vi "报告-报警采集 - 副本.vi"   [LabVIEW 2015]
uses:
  Global control/global-1.vi
  <userlib>/_OpenG.lib/array/array.llb/Search 1D Array (Boolean)__ogtk.vi
  Global control/global-2.vi
  Global control/global-opc.vi
types:
  T1 = cluster{"Host交流故障":bool, "Host交流缺相":bool, "Host交流失电":bool, "01#JLCL交流故障":bool, "01#JLCL交流缺相":bool, "01#JLCL交流失电":bool, "02#JLCL交流故障":bool, "02#JLCL交流缺相":bool, "02#JLCL交流失电":bool, "备用1":bool, "备用2":bool, "备用3":bool, "备用4":bool, "备用5":bool, "备用6":bool, " 备用7":bool}
  T2 = cluster{"09#电源模块故障":bool, "10#电源模块故障":bool, "11#电源模块故障":bool, "12#电源模块故障":bool, "13#电源模块故障":bool, "14#电源模块故障":bool, "15#电源模块故障":bool, "16#电源模块故障":bool, "01#电源模块故障":bool, "02#电源模块故障":bool, "03#电源模块故障":bool, "04#电源模块故障":bool, "05#电源模块故障":bool, "06#电源模块故障":bool, "07#电源模块故障":bool, " 08#电源模块故障":bool}
  T3 = cluster{"09#模块通信故障":bool, "10#模块通信故障":bool, "11#模块通信故障":bool, "12#模块通信故障":bool, "13#模块通信故障":bool, "14#模块通信故障":bool, "15#模块通信故障":bool, "16#模块通信故障":bool, "01#模块通信故障":bool, "02#模块通信故障":bool, "03#模块通信故障":bool, "04#模块通信故障":bool, "05#模块通信故障":bool, "06#模块通信故障":bool, "07#模块通信故障":bool, "08#模块通信故障":bool}
  T4 = cluster{"母线过压":bool, "母线欠压":bool, "母线绝缘异常":bool, "母线绝缘预警":bool, "母线绝缘压差故障":bool, "母线交流串入故障":bool, "备用5":bool, " 备用6":bool, "电池组过压":bool, "电池组欠压":bool, "电池组过温":bool, "单体电池故障":bool, "备用1":bool, "备用2":bool, "备用3":bool, " 备用4":bool}
  T5 = cluster{"合母输出3#告警":bool, "合母输出4#告警":bool, "合母输出5#告警":bool, "合母输出6#告警":bool, "13#开关状态":bool, "14#开关状态":bool, "15#开关状态":bool, "16#开关状态":bool, "控母输出1#告警":bool, "控母输出2#告警":bool, "控母输出3#告警":bool, "控母输出4#告警":bool, "控母输出5#告警":bool, "控母输出6#告警":bool, "合母输出1#告警":bool, "合母输出2#告警":bool}
  T6 = cluster{"25#开关状态":bool, "26#开关状态":bool, "27#开关状态":bool, "28#开关状态":bool, "29#开关状态":bool, "30#开关状态":bool, "31#开关状态":bool, "32#开关状态":bool, "交流输入I告警":bool, "交流输入II告警":bool, "19#开关状态":bool, "20#开关状态":bool, "21#开关状态":bool, "22#开关状态":bool, "23#开关状态":bool, "24#开关状态":bool}
  T7 = cluster{"动作报告1":bool, "动作报告2":bool, "动作报告3":bool, "动作报告4":bool, "动作报告5":bool, "动作报告6":bool, "动作报告7":bool, "动作报告8":bool, "动作报告9":bool, "动作报告10":bool, "动作报告11":bool, "动作报告12":bool, "动作报告13":bool, "动作报告14":bool, "动作报告15":bool, "动作报告16":bool, "重合闸成功":bool, "线路测试失败":bool, "重合闸失败":bool, "手动合闸失败":bool, "一次重合":bool, "二次重合":bool, "三次重合":bool, "四次重合":bool, "失灵保护跳闸":bool, "失灵保护重跳":bool}
  T8 = cluster{"动作信号":bool, "异常告警":bool, "断路器合闸位置":bool, "隔离开关合闸位置":bool, "远方就地（1就地）":bool, "扩展板异常告警":bool, "虚遥信7":bool, "虚遥信8":bool, "虚遥信9":bool, "虚遥信10":bool, "虚遥信11":bool, "虚遥信12":bool, "虚遥信13":bool, "虚遥信14":bool, "虚遥信15":bool, "虚遥信16":bool}
  T9 = cluster{"直接合闸":bool, "分闸复位":bool, "带测合闸":bool, "MCB故障":bool, "断路器合闸反馈信号":bool, "ED储能":bool, "应急分闸":bool, "断路器分闸反馈信号":bool, "远程控制":bool, "就地控制":bool, "试验位置":bool, "工作位置":bool, "带测接触器":bool, "本站框架":bool, "邻站过流":bool, "邻站框架":bool}
  T10 = cluster{"toHMI正常运行":bool, "toHMI异常跳闸":bool, "toHMI远程":bool, "toHMI模拟中压合闸—按钮":bool, "toHMI负极柜故障报警":bool, "toHMI正极柜故障报警":bool, "toHMI馈线柜故障报警":bool, "toHMI上网柜故障报警":bool, "toHMI整流柜故障报警":bool, "toHMI压敏快熔故障":bool, "toHMI整流柜跳闸":bool, "toHMI整流柜合闸—状态":bool, "直流电流输出":u32, "直流220V电压输出":u32, "380电压输入":u32, "模拟中压合闸控制":bool, "toHMI本地":bool}
  T11 = cluster{"toHMI正常运行":bool, "toHMI设备准备好":bool, "toHMI设备异常":bool, "toHMI刀开关合—状态":bool, "toHMI刀开关分—状态":bool, "toHMI刀开关合按钮":bool, "toHMI刀开关分按钮":bool, "toHMI复位按钮":bool, "toHMI远程":bool, "toHMI本地":bool, "toHMI刀闸合—动作":bool, "toHMI刀闸分—动作":bool, "刀开关合闸控制":bool, "刀开关分闸控制":bool, "故障复位控制":bool}
  T12 = cluster{"60":bool, "70":bool, "2120":bool, "212":bool, "2121":bool, "2124":bool, "214":bool, "2140":bool, "2141":bool, "90":bool, "2110":bool, "211":bool, "2111":bool, "2113":bool, "备用1":bool, "备用2":bool}
  T13 = cluster{"toHMI正常运行":bool, "toHMI设备准备好":bool, "toHMI设备异常":bool, "toHMI高断分—状态":bool, "toHMI高断合—状态":bool, "toHMI继保故障信号":bool, "toHMI远方":bool, "toHMI本地":bool, "toHMI旁路合闸—按钮":bool, "toHMI旁路分闸—按钮":bool, "toHMI允许高断合闸—状态":bool, "toHMI旁路合分闸—状态":bool, "1500V电压输出":u32, "高断储能控制":bool, "旁路合闸控制":bool, "旁路分闸控制":bool}
  T14 = cluster{"toHMI正常运行":bool, "toHMI设备准备好":bool, "toHMI设备异常":bool, "toHMI刀开关分—状态":bool, "toHMI刀开关合—状态":bool, "toHMI框架电流故障":bool, "toHMI框架电压故障":bool, "toHMII段电压故障":bool, "toHMIII段电压故障":bool, "toHMI装置故障":bool, "toHMIMCB故障":bool, "toHMI刀开关合—完成":bool, "toHMI复位按钮":bool, "toHMI远程":bool, "toHMI本地":bool, "模拟电流框架故障控制":bool, "模拟电压框架故障控制":bool, "模拟I段电压故障控制":bool, "模拟II段电压故障控制":bool, "故障复位控制":bool}
  T15 = cluster{"toHMI刀开关合—状态":bool, "toHMI刀开关分—状态":bool, "toHMI刀开关合按钮":bool, "toHMI刀开关分按钮":bool, "toHMI远程":bool, "toHMI本地":bool, "toHMI正常运行":bool, "toHMI设备准备好":bool, "toHMI设备异常":bool, "toHMI刀闸合—动作":bool, "toHMI刀闸分—动作":bool, "toHMI接触轨有压":bool, "刀开关合闸控制":bool, "刀开关分闸控制":bool}
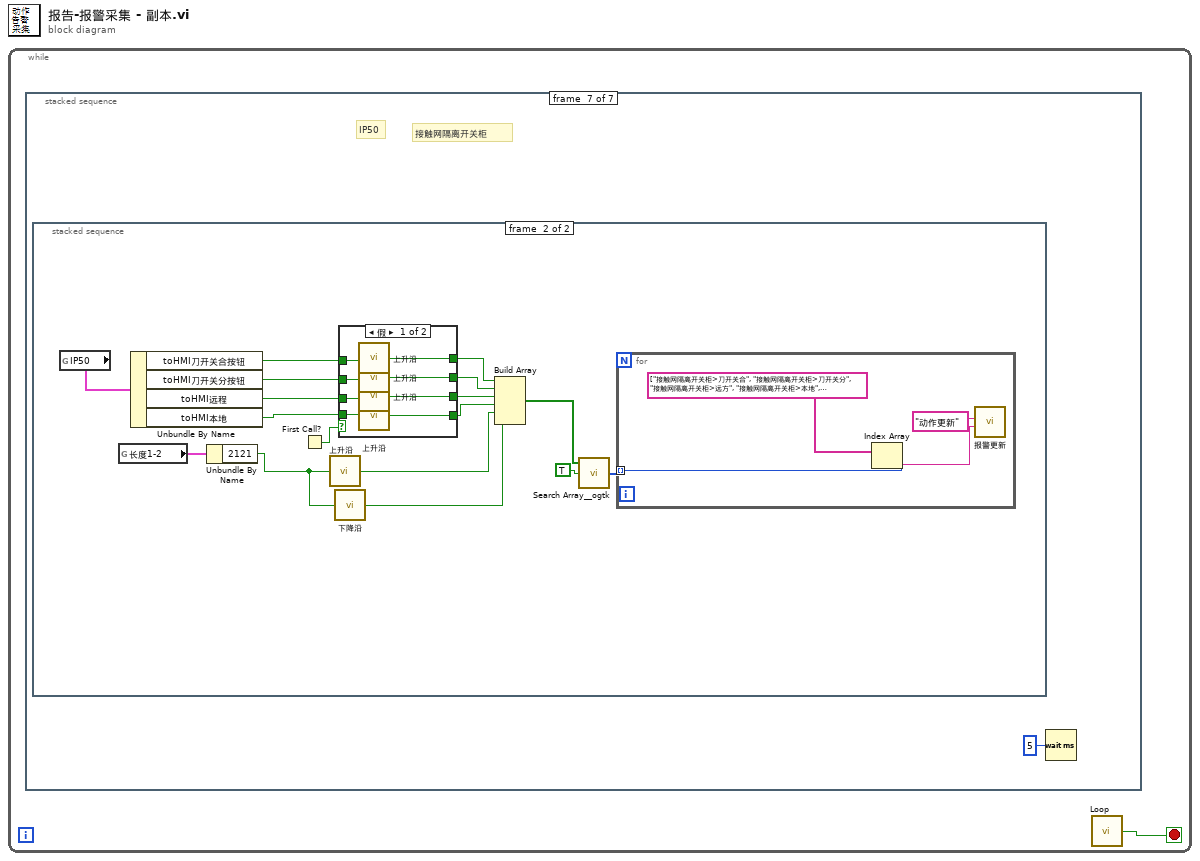
[diagram p0: block diagram]
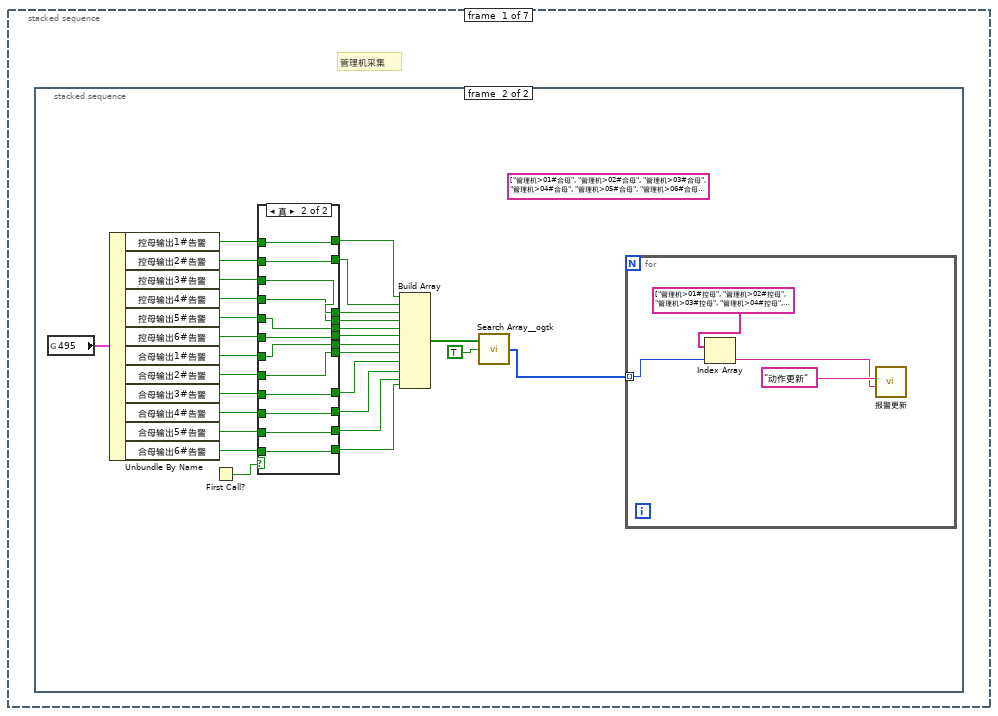
[diagram p2: hidden frame]
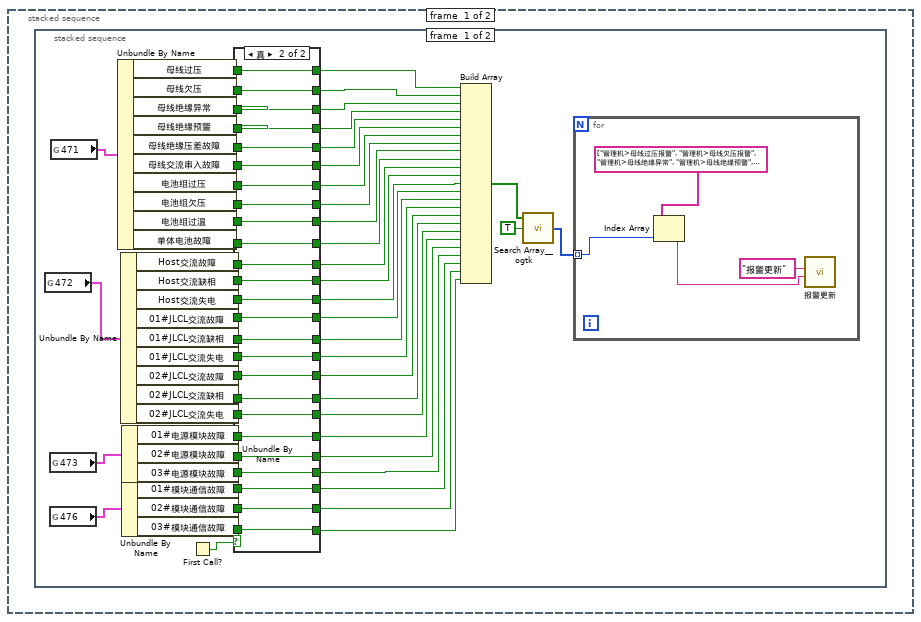
[diagram p3: hidden frame]
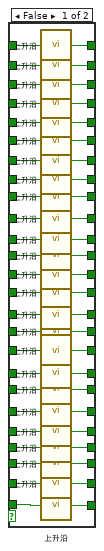
[diagram p4: hidden frame]
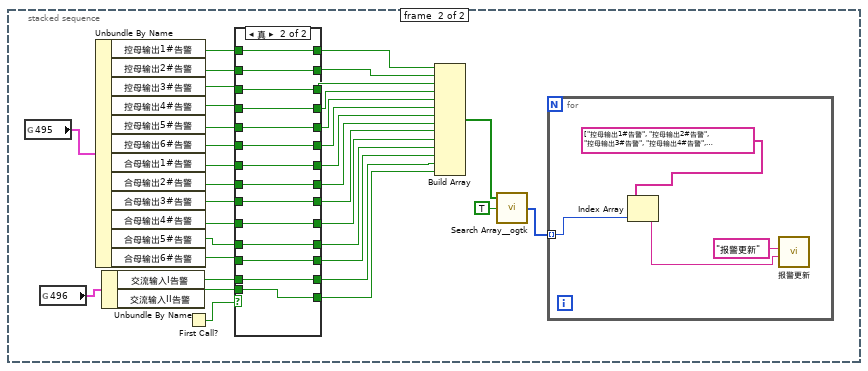
[diagram p5: hidden frame]
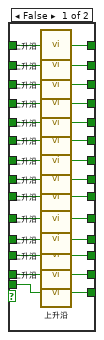
[diagram p6: hidden frame]
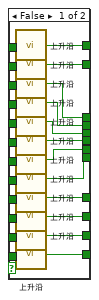
[diagram p7: hidden frame]
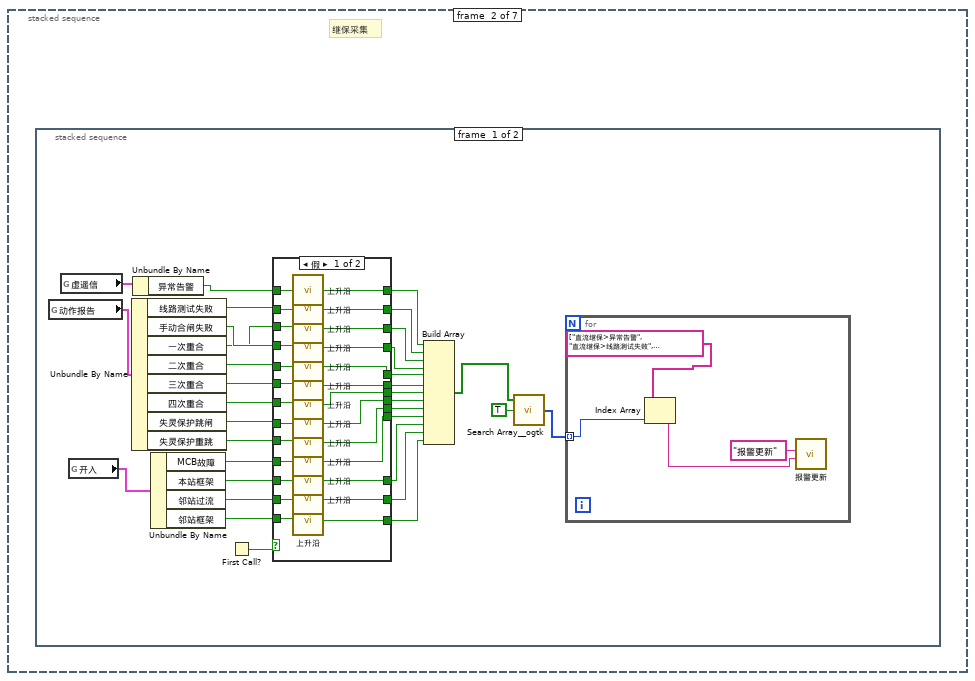
[diagram p8: hidden frame]
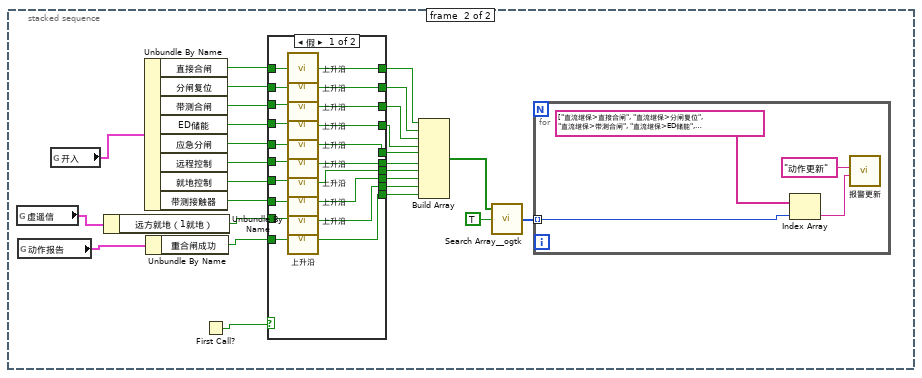
[diagram p10: hidden frame]
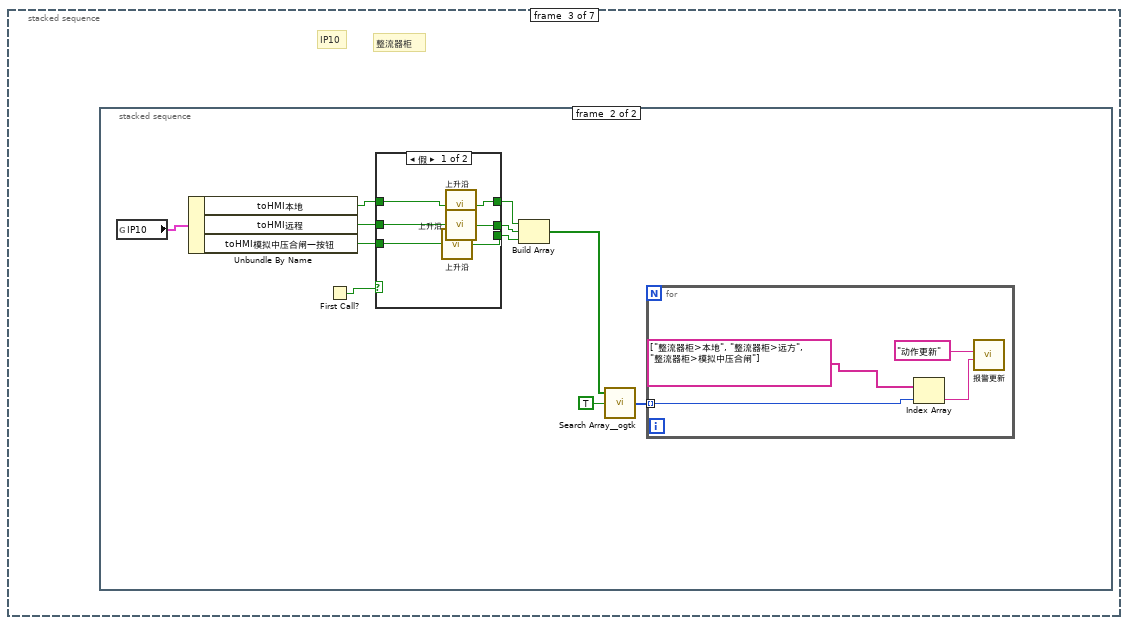
[diagram p12: hidden frame]
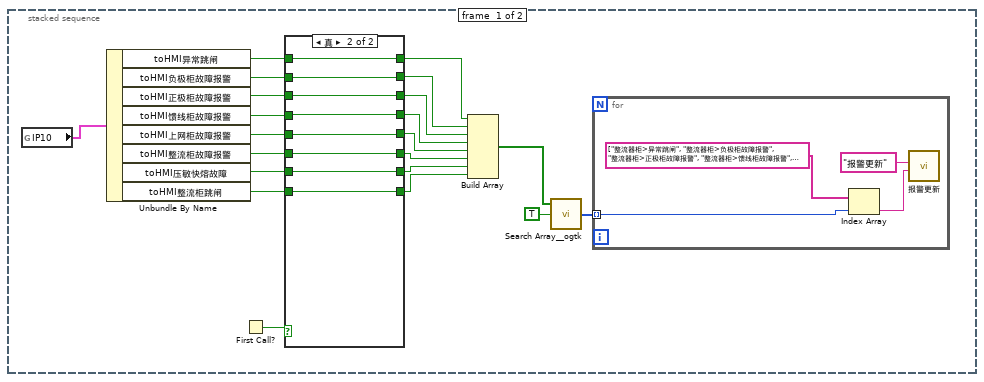
[diagram p13: hidden frame]
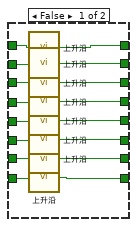
[diagram p14: hidden frame]
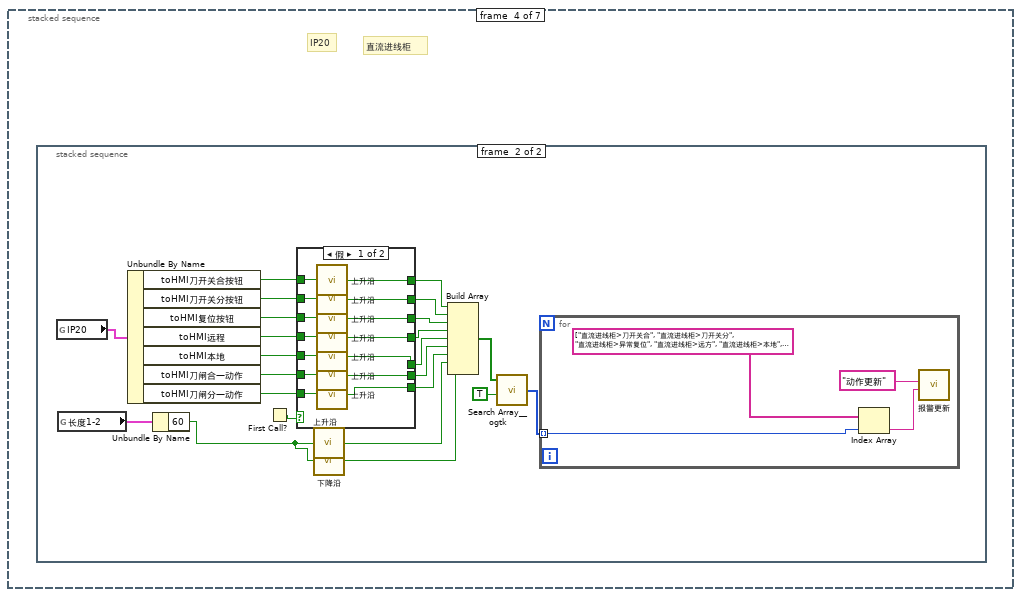
[diagram p16: hidden frame]
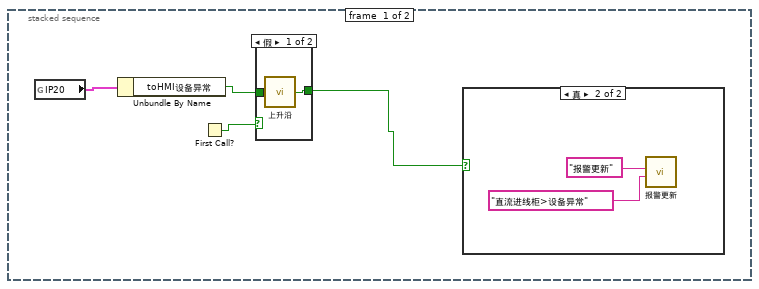
[diagram p17: hidden frame]
diagram:
  n1 = while {
    stop <- w1 stop-if-true
    n2 = stacked-sequence {
      frame #0 {
        # "管理机采集"
        n3 = stacked-sequence {
          frame #0 {
            n4 = stacked-sequence {
              frame #0 {
                n5 = global read "global-1.vi" "472"() -> (w58:T1)
                n6 = global read "global-1.vi" "473"() -> (w57:T2)
                n7 = global read "global-1.vi" "476"() -> (w56:T3)
                n8 = global read "global-1.vi" "471"() -> (w59:T4)
                n9 = Unbundle By Name(w59) -> ("母线过压"=w28:bool, "母线欠压"=w55:bool, "母线绝缘异常"=w54:bool, "母线绝缘预警"=w53:bool, "母线绝缘压差故障"=w52:bool, "母线交流串入故障"=w51:bool, "电池组过压"=w50:bool, "电池组欠压"=w49:bool, "电池组过温"=w48:bool, "单体电池故障"=w47:bool)
                n10 = Unbundle By Name(w58) -> ("Host交流故障"=w46:bool, "Host交流缺相"=w45:bool, "Host交流失电"=w44:bool, "01#JLCL交流故障"=w43:bool, "01#JLCL交流缺相"=w42:bool, "01#JLCL交流失电"=w41:bool, "02#JLCL交流故障"=w40:bool, "02#JLCL交流缺相"=w39:bool, "02#JLCL交流失电"=w38:bool)
                n11 = Unbundle By Name(w57) -> ("01#电源模块故障"=w37:bool, "02#电源模块故障"=w36:bool, "03#电源模块故障"=w35:bool)
                n12 = Unbundle By Name(w56) -> ("01#模块通信故障"=w34:bool, "02#模块通信故障"=w33:bool, "03#模块通信故障"=w32:bool)
                n13 = First Call?() -> (First Call?: T/F=w2:bool)
                n14 = case shown="真" w2 {
                  tunnel: w55 -> [w109 w133]
                  tunnel: w54 -> [w108 w132]
                  tunnel: w53 -> [w107 w131]
                  tunnel: w52 -> [w106 w130]
                  tunnel: w51 -> [w105 w129]
                  tunnel: w50 -> [w104 w128]
                  tunnel: w49 -> [w103 w127]
                  tunnel: w48 -> [w102 w126]
                  tunnel: w47 -> [w101 w125]
                  tunnel: w46 -> [w100 w124]
                  tunnel: w45 -> [w99 w123]
                  tunnel: w44 -> [w98 w122]
                  tunnel: w43 -> [w97 w121]
                  tunnel: w42 -> [w96 w120]
                  tunnel: w41 -> [w95 w119]
                  tunnel: w40 -> [w94 w118]
                  tunnel: w39 -> [w93 w117]
                  tunnel: w38 -> [w92 w116]
                  tunnel: w37 -> [w91 w115]
                  tunnel: w36 -> [w90 w114]
                  tunnel: w35 -> [w89 w113]
                  tunnel: w34 -> [w88 w112]
                  tunnel: w33 -> [w87 w111]
                  tunnel: w32 -> [w86 w110]
                  tunnel: w28 -> [w85 w134]
                  tunnel: [w84 w134] -> w27
                  tunnel: [w83 w133] -> w26
                  tunnel: [w82 w132] -> w25
                  tunnel: [w81 w131] -> w24
                  tunnel: [w80 w130] -> w23
                  tunnel: [w79 w129] -> w22
                  tunnel: [w78 w128] -> w21
                  tunnel: [w77 w127] -> w20
                  tunnel: [w76 w126] -> w19
                  tunnel: [w75 w125] -> w18
                  tunnel: [w74 w124] -> w17
                  tunnel: [w73 w123] -> w16
                  tunnel: [w72 w122] -> w15
                  tunnel: [w71 w121] -> w14
                  tunnel: [w70 w120] -> w13
                  tunnel: [w69 w118] -> w12
                  tunnel: [w68 w117] -> w11
                  tunnel: [w67 w116] -> w10
                  tunnel: [w66 w115] -> w9
                  tunnel: [w65 w114] -> w8
                  tunnel: [w64 w113] -> w7
                  tunnel: [w63 w112] -> w6
                  tunnel: [w62 w111] -> w5
                  tunnel: [w61 w110] -> w4
                  tunnel: [w60 w119] -> w3
                  frame False {
                    n15 = call "上升沿.vi"("Boolean Input"=w85) -> ("Rising Edge"=w84:bool)
                    n16 = call "上升沿.vi"("Boolean Input"=w109) -> ("Rising Edge"=w83:bool)
                    n17 = call "上升沿.vi"("Boolean Input"=w108) -> ("Rising Edge"=w82:bool)
                    n18 = call "上升沿.vi"("Boolean Input"=w107) -> ("Rising Edge"=w81:bool)
                    n19 = call "上升沿.vi"("Boolean Input"=w106) -> ("Rising Edge"=w80:bool)
                    n20 = call "上升沿.vi"("Boolean Input"=w105) -> ("Rising Edge"=w79:bool)
                    n21 = call "上升沿.vi"("Boolean Input"=w104) -> ("Rising Edge"=w78:bool)
                    n22 = call "上升沿.vi"("Boolean Input"=w103) -> ("Rising Edge"=w77:bool)
                    n23 = call "上升沿.vi"("Boolean Input"=w102) -> ("Rising Edge"=w76:bool)
                    n24 = call "上升沿.vi"("Boolean Input"=w101) -> ("Rising Edge"=w75:bool)
                    n25 = call "上升沿.vi"("Boolean Input"=w100) -> ("Rising Edge"=w74:bool)
                    n26 = call "上升沿.vi"("Boolean Input"=w99) -> ("Rising Edge"=w73:bool)
                    n27 = call "上升沿.vi"("Boolean Input"=w98) -> ("Rising Edge"=w72:bool)
                    n28 = call "上升沿.vi"("Boolean Input"=w97) -> ("Rising Edge"=w71:bool)
                    n29 = call "上升沿.vi"("Boolean Input"=w96) -> ("Rising Edge"=w70:bool)
                    n30 = call "上升沿.vi"("Boolean Input"=w95) -> ("Rising Edge"=w60:bool)
                    n31 = call "上升沿.vi"("Boolean Input"=w94) -> ("Rising Edge"=w69:bool)
                    n32 = call "上升沿.vi"("Boolean Input"=w93) -> ("Rising Edge"=w68:bool)
                    n33 = call "上升沿.vi"("Boolean Input"=w92) -> ("Rising Edge"=w67:bool)
                    n34 = call "上升沿.vi"("Boolean Input"=w91) -> ("Rising Edge"=w66:bool)
                    n35 = call "上升沿.vi"("Boolean Input"=w90) -> ("Rising Edge"=w65:bool)
                    n36 = call "上升沿.vi"("Boolean Input"=w89) -> ("Rising Edge"=w64:bool)
                    n37 = call "上升沿.vi"("Boolean Input"=w88) -> ("Rising Edge"=w63:bool)
                    n38 = call "上升沿.vi"("Boolean Input"=w87) -> ("Rising Edge"=w62:bool)
                    n39 = call "上升沿.vi"("Boolean Input"=w86) -> ("Rising Edge"=w61:bool)
                  }
                  frame True {
                  }
                }
                n40 = Build Array(w27, w26, w25, w24, w23, w22, w21, w20, w19, w18, w17, w16, w15, w14, w13, w3, w12, w11, w10, w9, w8, w7, w6, w5, w4) -> (w29:bool[])
                n41 = call-poly <userlib>:"Search Array__ogtk.vi"("Array"=w29, "Element Data"=TRUE) -> ("Indices of Elements"=w30:i32[])  [unwired: 7 in]
                n42 = for {
                  tunnel: w30 -> [w137] mode=indexing
                  n43 = Index Array(array=string[] ["管理机>母线过压报警", "管理机>母线欠压报警", "管理机>母线绝缘异常", "管理机>母线绝缘预警", "管理机>母线绝缘压差故障", "管理机>母线交流串入故障", "管理机>电池组过压", "管理机>电池组欠压", "管理机>电池组过温", "管理机>单体电池故障", "管理机>Host交流故障", "管理机>Host交流缺相", "管理机>Host交流失电", "管理机>01#JLCL交流故障", "管理机>01#JLCL交流缺相", "管理机>01#JLCL交流失电", "管理机>02#JLCL交流故障", "管理机>02#JLCL交流缺相", "管理机>02#JLCL交流失电", "管理机>01#电源模块故障", "管理机>02#电源模块故障", "管理机>03#电源模块故障", "管理机>01##模块通信故障", "管理机>02##模块通信故障", "管理机>03##模块通信故障"], index=w137) -> (element=w136:string)
                  n44 = call "报警更新.vi"("Message Data"=w136, "state"="报警更新") -> ()  [unwired: 10 in]
                }
              }
              frame #1 {
                n45 = global read "global-1.vi" "495"() -> (w172:T5)
                n46 = global read "global-1.vi" "496"() -> (w171:T6)
                n47 = Unbundle By Name(w172) -> ("控母输出1#告警"=w156:bool, "控母输出2#告警"=w170:bool, "控母输出3#告警"=w169:bool, "控母输出4#告警"=w168:bool, "控母输出5#告警"=w167:bool, "控母输出6#告警"=w166:bool, "合母输出1#告警"=w165:bool, "合母输出2#告警"=w164:bool, "合母输出3#告警"=w163:bool, "合母输出4#告警"=w162:bool, "合母输出5#告警"=w140:bool, "合母输出6#告警"=w139:bool)
                n48 = Unbundle By Name(w171) -> ("交流输入I告警"=w161:bool, "交流输入II告警"=w160:bool)
                n49 = First Call?() -> (First Call?: T/F=w141:bool)
                n50 = case shown="真" w141 {
                  tunnel: w170 -> [w200 w213]
                  tunnel: w169 -> [w199 w212]
                  tunnel: w168 -> [w198 w211]
                  tunnel: w167 -> [w197 w210]
                  tunnel: w166 -> [w196 w209]
                  tunnel: w165 -> [w195 w208]
                  tunnel: w164 -> [w194 w207]
                  tunnel: w163 -> [w193 w206]
                  tunnel: w162 -> [w192 w205]
                  tunnel: w140 -> [w191 w204]
                  tunnel: w139 -> [w190 w203]
                  tunnel: w161 -> [w189 w202]
                  tunnel: w160 -> [w188 w201]
                  tunnel: w156 -> [w187 w214]
                  tunnel: [w186 w214] -> w155
                  tunnel: [w185 w213] -> w154
                  tunnel: [w184 w212] -> w153
                  tunnel: [w183 w211] -> w152
                  tunnel: [w182 w210] -> w151
                  tunnel: [w181 w209] -> w150
                  tunnel: [w180 w208] -> w149
                  tunnel: [w179 w207] -> w148
                  tunnel: [w178 w206] -> w147
                  tunnel: [w177 w205] -> w146
                  tunnel: [w176 w204] -> w145
                  tunnel: [w175 w203] -> w144
                  tunnel: [w174 w202] -> w143
                  tunnel: [w173 w201] -> w142
                  frame False {
                    n51 = call "上升沿.vi"("Boolean Input"=w187) -> ("Rising Edge"=w186:bool)
                    n52 = call "上升沿.vi"("Boolean Input"=w200) -> ("Rising Edge"=w185:bool)
                    n53 = call "上升沿.vi"("Boolean Input"=w199) -> ("Rising Edge"=w184:bool)
                    n54 = call "上升沿.vi"("Boolean Input"=w198) -> ("Rising Edge"=w183:bool)
                    n55 = call "上升沿.vi"("Boolean Input"=w197) -> ("Rising Edge"=w182:bool)
                    n56 = call "上升沿.vi"("Boolean Input"=w196) -> ("Rising Edge"=w181:bool)
                    n57 = call "上升沿.vi"("Boolean Input"=w195) -> ("Rising Edge"=w180:bool)
                    n58 = call "上升沿.vi"("Boolean Input"=w194) -> ("Rising Edge"=w179:bool)
                    n59 = call "上升沿.vi"("Boolean Input"=w193) -> ("Rising Edge"=w178:bool)
                    n60 = call "上升沿.vi"("Boolean Input"=w192) -> ("Rising Edge"=w177:bool)
                    n61 = call "上升沿.vi"("Boolean Input"=w191) -> ("Rising Edge"=w176:bool)
                    n62 = call "上升沿.vi"("Boolean Input"=w190) -> ("Rising Edge"=w175:bool)
                    n63 = call "上升沿.vi"("Boolean Input"=w189) -> ("Rising Edge"=w174:bool)
                    n64 = call "上升沿.vi"("Boolean Input"=w188) -> ("Rising Edge"=w173:bool)
                  }
                  frame True {
                  }
                }
                n65 = Build Array(w155, w154, w153, w152, w151, w150, w149, w148, w147, w146, w145, w144, w143, w142) -> (w157:bool[])
                n66 = call-poly <userlib>:"Search Array__ogtk.vi"("Array"=w157, "Element Data"=TRUE) -> ("Indices of Elements"=w158:i32[])  [unwired: 7 in]
                n67 = for {
                  tunnel: w158 -> [w217] mode=indexing
                  n68 = Index Array(array=string[] ["控母输出1#告警", "控母输出2#告警", "控母输出3#告警", "控母输出4#告警", "控母输出5#告警", "控母输出6#告警", "合母输出1#告警", "合母输出2#告警", "合母输出3#告警", "合母输出4#告警", "合母输出5#告警", "合母输出6#告警", "交流输入I告警", "交流输入II告警"], index=w217) -> (element=w216:string)
                  n69 = call "报警更新.vi"("Message Data"=w216, "state"="报警更新") -> ()  [unwired: 10 in]
                }
              }
            }
          }
          frame #1 {
            (unwired) string[] ["管理机>01#合母", "管理机>02#合母", "管理机>03#合母", "管理机>04#合母", "管理机>05#合母", "管理机>06#合母", "管理机>01#控母", "管理机>02#控母", "管理机>03#控母", "管理机>04#控母", "管理机>05#控母", "管理机>06#控母"]
            n70 = global read "global-1.vi" "495"() -> (w235:T5)
            n71 = Unbundle By Name(w235) -> ("控母输出1#告警"=w247:bool, "控母输出2#告警"=w246:bool, "控母输出3#告警"=w245:bool, "控母输出4#告警"=w244:bool, "控母输出5#告警"=w243:bool, "控母输出6#告警"=w242:bool, "合母输出1#告警"=w241:bool, "合母输出2#告警"=w240:bool, "合母输出3#告警"=w239:bool, "合母输出4#告警"=w238:bool, "合母输出5#告警"=w237:bool, "合母输出6#告警"=w236:bool)
            n72 = First Call?() -> (First Call?: T/F=w219:bool)
            n73 = case shown="真" w219 {
              tunnel: w247 -> [w271 w283]
              tunnel: w246 -> [w270 w282]
              tunnel: w245 -> [w269 w281]
              tunnel: w244 -> [w268 w280]
              tunnel: w243 -> [w267 w279]
              tunnel: w242 -> [w266 w278]
              tunnel: w241 -> [w265 w277]
              tunnel: w240 -> [w264 w276]
              tunnel: w239 -> [w263 w275]
              tunnel: w238 -> [w262 w274]
              tunnel: w237 -> [w261 w273]
              tunnel: w236 -> [w260 w272]
              tunnel: [w259 w283] -> w234
              tunnel: [w258 w282] -> w233
              tunnel: [w257 w281] -> w232
              tunnel: [w256 w280] -> w231
              tunnel: [w255 w279] -> w230
              tunnel: [w254 w278] -> w229
              tunnel: [w253 w277] -> w228
              tunnel: [w252 w276] -> w227
              tunnel: [w251 w275] -> w226
              tunnel: [w250 w274] -> w225
              tunnel: [w249 w273] -> w224
              tunnel: [w248 w272] -> w223
              frame False {
                n74 = call "上升沿.vi"("Boolean Input"=w271) -> ("Rising Edge"=w259:bool)
                n75 = call "上升沿.vi"("Boolean Input"=w270) -> ("Rising Edge"=w258:bool)
                n76 = call "上升沿.vi"("Boolean Input"=w269) -> ("Rising Edge"=w257:bool)
                n77 = call "上升沿.vi"("Boolean Input"=w268) -> ("Rising Edge"=w256:bool)
                n78 = call "上升沿.vi"("Boolean Input"=w267) -> ("Rising Edge"=w255:bool)
                n79 = call "上升沿.vi"("Boolean Input"=w266) -> ("Rising Edge"=w254:bool)
                n80 = call "上升沿.vi"("Boolean Input"=w265) -> ("Rising Edge"=w253:bool)
                n81 = call "上升沿.vi"("Boolean Input"=w264) -> ("Rising Edge"=w252:bool)
                n82 = call "上升沿.vi"("Boolean Input"=w263) -> ("Rising Edge"=w251:bool)
                n83 = call "上升沿.vi"("Boolean Input"=w262) -> ("Rising Edge"=w250:bool)
                n84 = call "上升沿.vi"("Boolean Input"=w261) -> ("Rising Edge"=w249:bool)
                n85 = call "上升沿.vi"("Boolean Input"=w260) -> ("Rising Edge"=w248:bool)
              }
              frame True {
              }
            }
            n86 = Build Array(w234, w233, w232, w231, w230, w229, w228, w227, w226, w225, w224, w223) -> (w222:bool[])
            n87 = call-poly <userlib>:"Search Array__ogtk.vi"("Array"=w222, "Element Data"=TRUE) -> ("Indices of Elements"=w220:i32[])  [unwired: 7 in]
            n88 = for {
              tunnel: w220 -> [w286] mode=indexing
              n89 = Index Array(array=string[] ["管理机>01#控母", "管理机>02#控母", "管理机>03#控母", "管理机>04#控母", "管理机>05#控母", "管理机>06#控母", "管理机>01#合母", "管理机>02#合母", "管理机>03#合母", "管理机>04#合母", "管理机>05#合母", "管理机>06#合母"], index=w286) -> (element=w285:string)
              n90 = call "报警更新.vi"("Message Data"=w285, "state"="动作更新") -> ()  [unwired: 10 in]
            }
          }
        }
      }
      frame #1 {
        # "继保采集"
        n91 = stacked-sequence {
          frame #0 {
            n92 = global read "global-2.vi" "动作报告"() -> (w319:T7)
            n93 = global read "global-2.vi" "虚遥信"() -> (w320:T8)
            n94 = global read "global-2.vi" "开入"() -> (w318:T9)
            n95 = Unbundle By Name(w319) -> ("线路测试失败"=w304:bool, "手动合闸失败"=w289:bool, "一次重合"=w288:bool, "二次重合"=w303:bool, "三次重合"=w302:bool, "四次重合"=w301:bool, "失灵保护跳闸"=w300:bool, "失灵保护重跳"=w299:bool)
            n96 = Unbundle By Name(w320) -> ("异常告警"=w305:bool)
            n97 = Unbundle By Name(w318) -> ("MCB故障"=w298:bool, "本站框架"=w297:bool, "邻站过流"=w296:bool, "邻站框架"=w295:bool)
            n98 = First Call?() -> (First Call?: T/F=w293:bool)
            n99 = case shown="假" w293 {
              tunnel: [w350 w363] -> w317
              tunnel: [w349 w362] -> w316
              tunnel: [w348 w361] -> w315
              tunnel: [w347 w360] -> w314
              tunnel: [w346 w359] -> w313
              tunnel: [w345 w358] -> w312
              tunnel: [w344 w357] -> w311
              tunnel: [w343 w356] -> w310
              tunnel: [w342 w355] -> w309
              tunnel: [w341 w354] -> w308
              tunnel: [w340 w353] -> w307
              tunnel: [w339 w352] -> w306
              tunnel: w305 -> [w338 w363]
              tunnel: w304 -> [w337 w362]
              tunnel: w288 -> [w336 w361]
              tunnel: w289 -> [w335 w360]
              tunnel: w303 -> [w334 w359]
              tunnel: w302 -> [w333 w358]
              tunnel: w301 -> [w332 w357]
              tunnel: w300 -> [w331 w356]
              tunnel: w299 -> [w330 w355]
              tunnel: w298 -> [w329 w354]
              tunnel: w297 -> [w328 w353]
              tunnel: w296 -> [w327 w352]
              tunnel: w295 -> [w326 w351]
              tunnel: [w325 w351] -> w294
              frame False {
                n100 = call "上升沿.vi"("Boolean Input"=w338) -> ("Rising Edge"=w350:bool)
                n101 = call "上升沿.vi"("Boolean Input"=w337) -> ("Rising Edge"=w349:bool)
                n102 = call "上升沿.vi"("Boolean Input"=w336) -> ("Rising Edge"=w348:bool)
                n103 = call "上升沿.vi"("Boolean Input"=w335) -> ("Rising Edge"=w347:bool)
                n104 = call "上升沿.vi"("Boolean Input"=w334) -> ("Rising Edge"=w346:bool)
                n105 = call "上升沿.vi"("Boolean Input"=w333) -> ("Rising Edge"=w345:bool)
                n106 = call "上升沿.vi"("Boolean Input"=w332) -> ("Rising Edge"=w344:bool)
                n107 = call "上升沿.vi"("Boolean Input"=w331) -> ("Rising Edge"=w343:bool)
                n108 = call "上升沿.vi"("Boolean Input"=w330) -> ("Rising Edge"=w342:bool)
                n109 = call "上升沿.vi"("Boolean Input"=w329) -> ("Rising Edge"=w341:bool)
                n110 = call "上升沿.vi"("Boolean Input"=w328) -> ("Rising Edge"=w340:bool)
                n111 = call "上升沿.vi"("Boolean Input"=w327) -> ("Rising Edge"=w339:bool)
                n112 = call "上升沿.vi"("Boolean Input"=w326) -> ("Rising Edge"=w325:bool)
              }
              frame True {
              }
            }
            n113 = Build Array(w317, w316, w315, w314, w313, w312, w311, w310, w309, w308, w307, w306, w294) -> (w290:bool[])
            n114 = call-poly <userlib>:"Search Array__ogtk.vi"("Array"=w290, "Element Data"=TRUE) -> ("Indices of Elements"=w291:i32[])  [unwired: 7 in]
            n115 = for {
              tunnel: w291 -> [w323] mode=indexing
              n116 = Index Array(array=string[] ["直流继保>异常告警", "直流继保>线路测试失败", "直流继保>手动合闸失败", "直流继保>一次重合", "直流继保>二次重合", "直流继保>三次重合", "直流继保>四次重合", "直流继保>失灵保护跳闸", "直流继保>失灵保护重跳", "直流继保>MCB故障", "直流继保>本站框架", "直流继保>邻站过流", "直流继保>邻站框架"], index=w323) -> (element=w322:string)
              n117 = call "报警更新.vi"("Message Data"=w322, "state"="报警更新") -> ()  [unwired: 10 in]
            }
          }
          frame #1 {
            n118 = global read "global-2.vi" "虚遥信"() -> (w389:T8)
            n119 = global read "global-2.vi" "动作报告"() -> (w388:T7)
            n120 = global read "global-2.vi" "开入"() -> (w390:T9)
            n121 = Unbundle By Name(w389) -> ("远方就地（1就地）"=w369:bool)
            n122 = Unbundle By Name(w390) -> ("直接合闸"=w377:bool, "分闸复位"=w376:bool, "带测合闸"=w375:bool, "ED储能"=w374:bool, "应急分闸"=w373:bool, "远程控制"=w372:bool, "就地控制"=w371:bool, "带测接触器"=w370:bool)
            n123 = Unbundle By Name(w388) -> ("重合闸成功"=w368:bool)
            n124 = First Call?() -> (First Call?: T/F=w364:bool)
            n125 = case shown="假" w364 {
              tunnel: [w414 w424] -> w378
              tunnel: [w413 w423] -> w379
              tunnel: [w412 w422] -> w380
              tunnel: [w411 w421] -> w381
              tunnel: [w410 w420] -> w382
              tunnel: [w409 w419] -> w383
              tunnel: [w408 w418] -> w384
              tunnel: [w407 w417] -> w385
              tunnel: [w406 w416] -> w386
              tunnel: [w405 w415] -> w387
              tunnel: w377 -> [w404 w424]
              tunnel: w376 -> [w403 w423]
              tunnel: w375 -> [w402 w422]
              tunnel: w374 -> [w401 w421]
              tunnel: w373 -> [w400 w420]
              tunnel: w372 -> [w399 w419]
              tunnel: w371 -> [w398 w418]
              tunnel: w370 -> [w397 w417]
              tunnel: w369 -> [w396 w416]
              tunnel: w368 -> [w395 w415]
              frame False {
                n126 = call "上升沿.vi"("Boolean Input"=w404) -> ("Rising Edge"=w414:bool)
                n127 = call "上升沿.vi"("Boolean Input"=w403) -> ("Rising Edge"=w413:bool)
                n128 = call "上升沿.vi"("Boolean Input"=w402) -> ("Rising Edge"=w412:bool)
                n129 = call "上升沿.vi"("Boolean Input"=w401) -> ("Rising Edge"=w411:bool)
                n130 = call "上升沿.vi"("Boolean Input"=w400) -> ("Rising Edge"=w410:bool)
                n131 = call "上升沿.vi"("Boolean Input"=w399) -> ("Rising Edge"=w409:bool)
                n132 = call "上升沿.vi"("Boolean Input"=w398) -> ("Rising Edge"=w408:bool)
                n133 = call "上升沿.vi"("Boolean Input"=w397) -> ("Rising Edge"=w407:bool)
                n134 = call "上升沿.vi"("Boolean Input"=w396) -> ("Rising Edge"=w406:bool)
                n135 = call "上升沿.vi"("Boolean Input"=w395) -> ("Rising Edge"=w405:bool)
              }
              frame True {
              }
            }
            n136 = Build Array(w378, w379, w380, w381, w382, w383, w384, w385, w386, w387) -> (w365:bool[])
            n137 = call-poly <userlib>:"Search Array__ogtk.vi"("Array"=w365, "Element Data"=TRUE) -> ("Indices of Elements"=w366:i32[])  [unwired: 7 in]
            n138 = for {
              tunnel: w366 -> [w393] mode=indexing
              n139 = Index Array(array=string[] ["直流继保>直接合闸", "直流继保>分闸复位", "直流继保>带测合闸", "直流继保>ED储能", "直流继保>应急分闸", "直流继保>远方", "直流继保>本地", "直流继保>带测接触器", "直流继保>远方就地（1就地）", "直流继保>重合闸成功"], index=w393) -> (element=w392:string)
              n140 = call "报警更新.vi"("Message Data"=w392, "state"="动作更新") -> ()  [unwired: 10 in]
            }
          }
        }
      }
      frame #2 {
        # "整流器柜"
        # "IP10"
        n141 = stacked-sequence {
          frame #0 {
            n142 = global read "global-opc.vi" "IP10"() -> (w445:T10)
            n143 = Unbundle By Name(w445) -> ("toHMI异常跳闸"=w426:bool, "toHMI负极柜故障报警"=w436:bool, "toHMI正极柜故障报警"=w435:bool, "toHMI馈线柜故障报警"=w434:bool, "toHMI上网柜故障报警"=w433:bool, "toHMI整流柜故障报警"=w432:bool, "toHMI压敏快熔故障"=w431:bool, "toHMI整流柜跳闸"=w430:bool)
            n144 = First Call?() -> (First Call?: T/F=w444:bool)
            n145 = case shown="真" w444 {
              tunnel: [w465 w473] -> w437
              tunnel: [w452 w472] -> w438
              tunnel: [w464 w471] -> w439
              tunnel: [w463 w470] -> w440
              tunnel: [w462 w469] -> w441
              tunnel: [w461 w468] -> w442
              tunnel: [w460 w467] -> w443
              tunnel: w436 -> [w459 w473]
              tunnel: w435 -> [w458 w472]
              tunnel: w434 -> [w457 w471]
              tunnel: w433 -> [w456 w470]
              tunnel: w432 -> [w455 w469]
              tunnel: w431 -> [w454 w468]
              tunnel: w430 -> [w453 w467]
              tunnel: w426 -> [w451 w466]
              tunnel: [w450 w466] -> w425
              frame False {
                n146 = call "上升沿.vi"("Boolean Input"=w451) -> ("Rising Edge"=w450:bool)
                n147 = call "上升沿.vi"("Boolean Input"=w459) -> ("Rising Edge"=w465:bool)
                n148 = call "上升沿.vi"("Boolean Input"=w458) -> ("Rising Edge"=w452:bool)
                n149 = call "上升沿.vi"("Boolean Input"=w457) -> ("Rising Edge"=w464:bool)
                n150 = call "上升沿.vi"("Boolean Input"=w456) -> ("Rising Edge"=w463:bool)
                n151 = call "上升沿.vi"("Boolean Input"=w455) -> ("Rising Edge"=w462:bool)
                n152 = call "上升沿.vi"("Boolean Input"=w454) -> ("Rising Edge"=w461:bool)
                n153 = call "上升沿.vi"("Boolean Input"=w453) -> ("Rising Edge"=w460:bool)
              }
              frame True {
              }
            }
            n154 = Build Array(w425, w437, w438, w439, w440, w441, w442, w443) -> (w427:bool[])
            n155 = call-poly <userlib>:"Search Array__ogtk.vi"("Array"=w427, "Element Data"=TRUE) -> ("Indices of Elements"=w428:i32[])  [unwired: 7 in]
            n156 = for {
              tunnel: w428 -> [w448] mode=indexing
              n157 = Index Array(array=string[] ["整流器柜>异常跳闸", "整流器柜>负极柜故障报警", "整流器柜>正极柜故障报警", "整流器柜>馈线柜故障报警", "整流器柜>隔离开关柜故障报警", "整流器柜>故障报警", "整流器柜>压敏快熔故障", "整流器柜>跳闸"], index=w448) -> (element=w447:string)
              n158 = call "报警更新.vi"("Message Data"=w447, "state"="报警更新") -> ()  [unwired: 10 in]
            }
          }
          frame #1 {
            n159 = global read "global-opc.vi" "IP10"() -> (w484:T10)
            n160 = Unbundle By Name(w484) -> ("toHMI本地"=w474:bool, "toHMI远程"=w482:bool, "toHMI模拟中压合闸—按钮"=w483:bool)
            n161 = First Call?() -> (First Call?: T/F=w476:bool)
            n162 = case shown="假" w476 {
              tunnel: w483 -> [w490 w493]
              tunnel: w482 -> [w487 w492]
              tunnel: [w489 w492] -> w481
              tunnel: [w488 w493] -> w480
              tunnel: [w485 w491] -> w475
              tunnel: w474 -> [w486 w491]
              frame False {
                n163 = call "上升沿.vi"("Boolean Input"=w490) -> ("Rising Edge"=w488:bool)
                n164 = call "上升沿.vi"("Boolean Input"=w486) -> ("Rising Edge"=w485:bool)
                n165 = call "上升沿.vi"("Boolean Input"=w487) -> ("Rising Edge"=w489:bool)
              }
              frame True {
              }
            }
            n166 = Build Array(w475, w481, w480) -> (w477:bool[])
            n167 = call-poly <userlib>:"Search Array__ogtk.vi"("Array"=w477, "Element Data"=TRUE) -> ("Indices of Elements"=w478:i32[])  [unwired: 7 in]
            n168 = for {
              tunnel: w478 -> [w496] mode=indexing
              n169 = Index Array(array=string[] ["整流器柜>本地", "整流器柜>远方", "整流器柜>模拟中压合闸"], index=w496) -> (element=w495:string)
              n170 = call "报警更新.vi"("Message Data"=w495, "state"="动作更新") -> ()  [unwired: 10 in]
            }
          }
        }
      }
      frame #3 {
        # "直流进线柜"
        # "IP20"
        n171 = stacked-sequence {
          frame #0 {
            n172 = global read "global-opc.vi" "IP20"() -> (w501:T11)
            n173 = Unbundle By Name(w501) -> ("toHMI设备异常"=w500:bool)
            n174 = First Call?() -> (First Call?: T/F=w499:bool)
            n175 = case shown="假" w499 {
              tunnel: w500 -> [w505 w506]
              tunnel: [w504 w506] -> w498
              frame False {
                n176 = call "上升沿.vi"("Boolean Input"=w505) -> ("Rising Edge"=w504:bool)
              }
              frame True {
              }
            }
            n177 = case shown="真" w498 {
              frame False {
              }
              frame True {
                n178 = call "报警更新.vi"("Message Data"="直流进线柜>设备异常" ("字符串"), "state"="报警更新") -> ()  [unwired: 10 in]
              }
            }
          }
          frame #1 {
            n179 = global read "global-opc.vi" "IP20"() -> (w529:T11)
            n180 = global read "global-1.vi" "长度1-2"() -> (w510:T12)
            n181 = Unbundle By Name(w529) -> ("toHMI刀开关合按钮"=w518:bool, "toHMI刀开关分按钮"=w517:bool, "toHMI复位按钮"=w516:bool, "toHMI远程"=w515:bool, "toHMI本地"=w514:bool, "toHMI刀闸合—动作"=w513:bool, "toHMI刀闸分—动作"=w512:bool)
            n182 = Unbundle By Name(w510) -> ("60"=w509:bool)
            n183 = First Call?() -> (First Call?: T/F=w526:bool)
            n184 = case shown="假" w526 {
              tunnel: [w543 w550] -> w519
              tunnel: [w542 w549] -> w520
              tunnel: [w541 w548] -> w521
              tunnel: [w540 w547] -> w522
              tunnel: [w539 w546] -> w523
              tunnel: [w538 w545] -> w524
              tunnel: [w537 w544] -> w525
              tunnel: w518 -> [w536 w550]
              tunnel: w517 -> [w535 w549]
              tunnel: w516 -> [w534 w548]
              tunnel: w515 -> [w533 w547]
              tunnel: w514 -> [w532 w546]
              tunnel: w513 -> [w531 w545]
              tunnel: w512 -> [w530 w544]
              frame False {
                n185 = call "上升沿.vi"("Boolean Input"=w536) -> ("Rising Edge"=w543:bool)
                n186 = call "上升沿.vi"("Boolean Input"=w535) -> ("Rising Edge"=w542:bool)
                n187 = call "上升沿.vi"("Boolean Input"=w534) -> ("Rising Edge"=w541:bool)
                n188 = call "上升沿.vi"("Boolean Input"=w533) -> ("Rising Edge"=w540:bool)
                n189 = call "上升沿.vi"("Boolean Input"=w532) -> ("Rising Edge"=w539:bool)
                n190 = call "上升沿.vi"("Boolean Input"=w531) -> ("Rising Edge"=w538:bool)
                n191 = call "上升沿.vi"("Boolean Input"=w530) -> ("Rising Edge"=w537:bool)
              }
              frame True {
              }
            }
            n192 = call "上升沿.vi"("Boolean Input"=w509) -> ("Rising Edge"=w508:bool)
            n193 = call "下降沿.vi"("Boolean Input"=w509) -> ("Falling Edge"=w507:bool)
            n194 = Build Array(w519, w520, w521, w522, w523, w524, w525, w508, w507) -> (w511:bool[])
            n195 = call-poly <userlib>:"Search Array__ogtk.vi"("Array"=w511, "Element Data"=TRUE) -> ("Indices of Elements"=w527:i32[])  [unwired: 7 in]
            n196 = for {
              tunnel: w527 -> [w553] mode=indexing
              n197 = Index Array(array=string[] ["直流进线柜>刀开关合", "直流进线柜>刀开关分", "直流进线柜>异常复位", "直流进线柜>远方", "直流进线柜>本地", "直流进线柜>刀闸合", "直流进线柜>刀闸分", "直流进线柜>刀闸合", "直流进线柜>刀闸分"], index=w553) -> (element=w552:string)
              n198 = call "报警更新.vi"("Message Data"=w552, "state"="动作更新") -> ()  [unwired: 10 in]
            }
          }
        }
      }
      frame #4 {
        # "直流馈线柜"
        # "IP30"
        n199 = stacked-sequence {
          frame #0 {
            n200 = global read "global-opc.vi" "IP30"() -> (w563:T13)
            n201 = Unbundle By Name(w563) -> ("toHMI设备异常"=w559:bool, "toHMI继保故障信号"=w558:bool)
            n202 = First Call?() -> (First Call?: T/F=w562:bool)
            n203 = case shown="真" w562 {
              tunnel: [w571 w573] -> w560
              tunnel: [w570 w572] -> w561
              tunnel: w559 -> [w569 w573]
              tunnel: w558 -> [w568 w572]
              frame False {
                n204 = call "上升沿.vi"("Boolean Input"=w569) -> ("Rising Edge"=w571:bool)
                n205 = call "上升沿.vi"("Boolean Input"=w568) -> ("Rising Edge"=w570:bool)
              }
              frame True {
              }
            }
            n206 = Build Array(w560, w561) -> (w555:bool[])
            n207 = call-poly <userlib>:"Search Array__ogtk.vi"("Array"=w555, "Element Data"=TRUE) -> ("Indices of Elements"=w556:i32[])  [unwired: 7 in]
            n208 = for {
              tunnel: w556 -> [w566] mode=indexing
              n209 = Index Array(array=string[] ["直流馈线柜>设备异常", "直流馈线柜>继保故障信号"], index=w566) -> (element=w565:string)
              n210 = call "报警更新.vi"("Message Data"=w565, "state"="报警更新") -> ()  [unwired: 10 in]
            }
          }
          frame #1 {
            n211 = global read "global-opc.vi" "IP30"() -> (w586:T13)
            n212 = Unbundle By Name(w586) -> ("toHMI远方"=w580:bool, "toHMI本地"=w579:bool, "toHMI旁路合闸—按钮"=w578:bool, "toHMI旁路分闸—按钮"=w577:bool)
            n213 = First Call?() -> (First Call?: T/F=w585:bool)
            n214 = case shown="真" w585 {
              tunnel: [w598 w602] -> w581
              tunnel: [w597 w601] -> w582
              tunnel: [w596 w600] -> w583
              tunnel: [w595 w599] -> w584
              tunnel: w580 -> [w594 w602]
              tunnel: w579 -> [w593 w601]
              tunnel: w578 -> [w592 w600]
              tunnel: w577 -> [w591 w599]
              frame False {
                n215 = call "上升沿.vi"("Boolean Input"=w594) -> ("Rising Edge"=w598:bool)
                n216 = call "上升沿.vi"("Boolean Input"=w593) -> ("Rising Edge"=w597:bool)
                n217 = call "上升沿.vi"("Boolean Input"=w592) -> ("Rising Edge"=w596:bool)
                n218 = call "上升沿.vi"("Boolean Input"=w591) -> ("Rising Edge"=w595:bool)
              }
              frame True {
              }
            }
            n219 = Build Array(w581, w582, w583, w584) -> (w574:bool[])
            n220 = call-poly <userlib>:"Search Array__ogtk.vi"("Array"=w574, "Element Data"=TRUE) -> ("Indices of Elements"=w575:i32[])  [unwired: 7 in]
            n221 = for {
              tunnel: w575 -> [w589] mode=indexing
              n222 = Index Array(array=string[] ["直流馈线柜>远方", "直流馈线柜>本地", "直流馈线柜>旁路合闸", "直流馈线柜>旁路分闸"], index=w589) -> (element=w588:string)
              n223 = call "报警更新.vi"("Message Data"=w588, "state"="动作更新") -> ()  [unwired: 10 in]
            }
          }
        }
      }
      frame #5 {
        # "负极柜"
        # "IP40"
        n224 = stacked-sequence {
          frame #0 {
            (unwired) string[] ["负极柜>设备异常", "负极柜>框架电流故障", "负极柜>框架电压故障", "负极柜>I段电压故障", "负极柜>II段电压故障", "负极柜>MCB故障"]
            n225 = global read "global-opc.vi" "IP40"() -> (w621:T14)
            n226 = Unbundle By Name(w621) -> ("toHMI设备异常"=w614:bool, "toHMI框架电流故障"=w613:bool, "toHMI框架电压故障"=w612:bool, "toHMII段电压故障"=w611:bool, "toHMIII段电压故障"=w610:bool, "toHMI装置故障"=w609:bool, "toHMIMCB故障"=w608:bool)
            n227 = First Call?() -> (First Call?: T/F=w620:bool)
            n228 = case shown="真" w620 {
              tunnel: [w639 w646] -> w615
              tunnel: [w638 w645] -> w616
              tunnel: [w637 w644] -> w617
              tunnel: [w636 w643] -> w618
              tunnel: [w635 w642] -> w619
              tunnel: [w627 w641] -> w607
              tunnel: w614 -> [w634 w646]
              tunnel: w613 -> [w633 w645]
              tunnel: w612 -> [w632 w644]
              tunnel: w611 -> [w631 w643]
              tunnel: w610 -> [w630 w642]
              tunnel: w609 -> [w629 w641]
              tunnel: w608 -> [w628 w640]
              tunnel: [w626 w640] -> w606
              frame False {
                n229 = call "上升沿.vi"("Boolean Input"=w629) -> ("Rising Edge"=w627:bool)
                n230 = call "上升沿.vi"("Boolean Input"=w634) -> ("Rising Edge"=w639:bool)
                n231 = call "上升沿.vi"("Boolean Input"=w633) -> ("Rising Edge"=w638:bool)
                n232 = call "上升沿.vi"("Boolean Input"=w632) -> ("Rising Edge"=w637:bool)
                n233 = call "上升沿.vi"("Boolean Input"=w631) -> ("Rising Edge"=w636:bool)
                n234 = call "上升沿.vi"("Boolean Input"=w630) -> ("Rising Edge"=w635:bool)
                n235 = call "上升沿.vi"("Boolean Input"=w628) -> ("Rising Edge"=w626:bool)
              }
              frame True {
              }
            }
            n236 = Build Array(w615, w616, w617, w618, w619, w607, w606) -> (w603:bool[])
            n237 = call-poly <userlib>:"Search Array__ogtk.vi"("Array"=w603, "Element Data"=TRUE) -> ("Indices of Elements"=w604:i32[])  [unwired: 7 in]
            n238 = for {
              tunnel: w604 -> [w624] mode=indexing
              n239 = Index Array(array=string[] ["直流进线柜>设备异常", "直流进线柜>框架电流故障", "直流进线柜>框架电压故障", "直流进线柜>I段电压故障", "直流进线柜>II段电压故障", "直流进线柜>装置故障", "直流进线柜>MCB故障"], index=w624) -> (element=w623:string)
              n240 = call "报警更新.vi"("Message Data"=w623, "state"="报警更新") -> ()  [unwired: 10 in]
            }
          }
          frame #1 {
            n241 = global read "global-opc.vi" "IP40"() -> (w659:T14)
            n242 = Unbundle By Name(w659) -> ("toHMI刀开关合—完成"=w653:bool, "toHMI复位按钮"=w652:bool, "toHMI远程"=w651:bool, "toHMI本地"=w650:bool)
            n243 = First Call?() -> (First Call?: T/F=w658:bool)
            n244 = case shown="假" w658 {
              tunnel: [w671 w675] -> w654
              tunnel: [w670 w674] -> w655
              tunnel: [w669 w673] -> w656
              tunnel: [w668 w672] -> w657
              tunnel: w653 -> [w667 w675]
              tunnel: w652 -> [w666 w674]
              tunnel: w651 -> [w665 w673]
              tunnel: w650 -> [w664 w672]
              frame False {
                n245 = call "上升沿.vi"("Boolean Input"=w667) -> ("Rising Edge"=w671:bool)
                n246 = call "上升沿.vi"("Boolean Input"=w666) -> ("Rising Edge"=w670:bool)
                n247 = call "上升沿.vi"("Boolean Input"=w665) -> ("Rising Edge"=w669:bool)
                n248 = call "上升沿.vi"("Boolean Input"=w664) -> ("Rising Edge"=w668:bool)
              }
              frame True {
              }
            }
            n249 = Build Array(w654, w655, w656, w657) -> (w647:bool[])
            n250 = call-poly <userlib>:"Search Array__ogtk.vi"("Array"=w647, "Element Data"=TRUE) -> ("Indices of Elements"=w648:i32[])  [unwired: 7 in]
            n251 = for {
              tunnel: w648 -> [w662] mode=indexing
              n252 = Index Array(array=string[] ["负极柜>刀开关合完成", "负极柜>异常复位", "负极柜>远方", "负极柜>本地"], index=w662) -> (element=w661:string)
              n253 = call "报警更新.vi"("Message Data"=w661, "state"="动作更新") -> ()  [unwired: 10 in]
            }
          }
        }
      }
      frame #6 {
        # "接触网隔离开关柜"
        # "IP50"
        n254 = stacked-sequence {
          frame #0 {
            n255 = global read "global-opc.vi" "IP50"() -> (w680:T15)
            n256 = Unbundle By Name(w680) -> ("toHMI设备异常"=w679:bool)
            n257 = First Call?() -> (First Call?: T/F=w678:bool)
            n258 = case shown="真" w678 {
              tunnel: w679 -> [w684 w685]
              tunnel: [w683 w685] -> w677
              frame False {
                n259 = call "上升沿.vi"("Boolean Input"=w684) -> ("Rising Edge"=w683:bool)
              }
              frame True {
              }
            }
            n260 = case shown="真" w677 {
              frame False {
              }
              frame True {
                n261 = call "报警更新.vi"("Message Data"="接触网隔离开关柜>设备异常" ("字符串"), "state"="报警更新") -> ()  [unwired: 10 in]
              }
            }
          }
          frame #1 {
            n262 = global read "global-opc.vi" "IP50"() -> (w702:T15)
            n263 = global read "global-1.vi" "长度1-2"() -> (w689:T12)
            n264 = Unbundle By Name(w702) -> ("toHMI刀开关合按钮"=w696:bool, "toHMI刀开关分按钮"=w695:bool, "toHMI远程"=w694:bool, "toHMI本地"=w693:bool)
            n265 = Unbundle By Name(w689) -> ("2121"=w688:bool)
            n266 = First Call?() -> (First Call?: T/F=w701:bool)
            n267 = call "上升沿.vi"("Boolean Input"=w688) -> ("Rising Edge"=w687:bool)
            n268 = call "下降沿.vi"("Boolean Input"=w688) -> ("Falling Edge"=w686:bool)
            n269 = case shown="假" w701 {
              tunnel: [w714 w718] -> w697
              tunnel: [w713 w717] -> w698
              tunnel: [w712 w716] -> w699
              tunnel: [w711 w715] -> w700
              tunnel: w696 -> [w710 w718]
              tunnel: w695 -> [w709 w717]
              tunnel: w694 -> [w708 w716]
              tunnel: w693 -> [w707 w715]
              frame False {
                n270 = call "上升沿.vi"("Boolean Input"=w710) -> ("Rising Edge"=w714:bool)
                n271 = call "上升沿.vi"("Boolean Input"=w709) -> ("Rising Edge"=w713:bool)
                n272 = call "上升沿.vi"("Boolean Input"=w708) -> ("Rising Edge"=w712:bool)
                n273 = call "上升沿.vi"("Boolean Input"=w707) -> ("Rising Edge"=w711:bool)
              }
              frame True {
              }
            }
            n274 = Build Array(w697, w698, w699, w700, w687, w686) -> (w690:bool[])
            n275 = call-poly <userlib>:"Search Array__ogtk.vi"("Array"=w690, "Element Data"=TRUE) -> ("Indices of Elements"=w691:i32[])  [unwired: 7 in]
            n276 = for {
              tunnel: w691 -> [w705] mode=indexing
              n277 = Index Array(array=string[] ["接触网隔离开关柜>刀开关合", "接触网隔离开关柜>刀开关分", "接触网隔离开关柜>远方", "接触网隔离开关柜>本地", "接触网隔离开关柜>刀开关合", "接触网隔离开关柜>刀开关分"], index=w705) -> (element=w704:string)
              n278 = call "报警更新.vi"("Message Data"=w704, "state"="动作更新") -> ()  [unwired: 10 in]
            }
          }
        }
        n279 = Wait (ms)(milliseconds to wait=u32 5 ("等待时间（毫秒）")) -> ()  [unwired: 1 out]
      }
    }
    n280 = call "Loop.vi"() -> ("Loop Out"=w1:bool)  [unwired: 5 in]
  }
